vi "Generate Day Start And Day End Times.vi"(11 "Day":timestamp) -> (2 "Day End":timestamp, 3 "Day Start":timestamp)   [LabVIEW 2015, in "Utility.lvlib"]
uses:
  Utility.lvlib
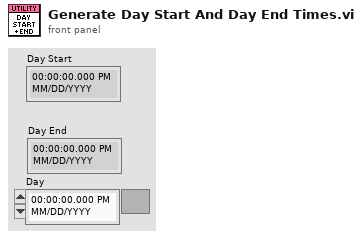
[diagram p1: front panel]
types:
  T1 = typedef "LVDateTimeRec.ctl" = cluster{"fractional second":dbl, "second":i32, "minute":i32, "hour":i32, "day of month":i32, "month":i32, "year":i32, "day of week":i32, "day of year":i32, "DST":i32}
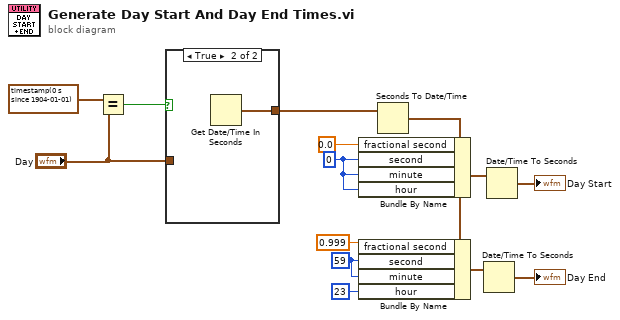
[diagram p0: block diagram]
diagram:
  w9 = 59 ("second")
  w13 = 0 ("second")
  n1 = Equal?(x=timestamp(0 s since 1904-01-01) ("current time"), y="Day") -> (x = y?=w3:bool)
  n2 = case shown="True" w3 {
    tunnel: [w15 w16] -> w14
    tunnel: "Day" -> [w15 _]
    frame False {
    }
    frame True {
      n3 = Get Date/Time In Seconds() -> (seconds since 1Jan1904=w16:timestamp)
    }
  }
  n4 = Seconds To Date/Time(time stamp (now)=w14) -> (date time rec=w10:T1)  [unwired: 1 in]
  n5 = Bundle By Name(cluster=w10, "fractional second"=0.0, "second"=w13, "minute"=w13, "hour"=w13) -> (w12:T1)
  n6 = Bundle By Name(cluster=w10, "fractional second"=0.999, "second"=w9, "minute"=w9, "hour"=23 ("second")) -> (w7:T1)
  n7 = Date/Time To Seconds(2:w7) -> (0:→"Day End":timestamp)  [unwired: 1 in]
  n8 = Date/Time To Seconds(2:w12) -> (0:→"Day Start":timestamp)  [unwired: 1 in]
